vi "Routine.vi"(11 "Base Event in":refnum<class "Base Event.lvclass">) -> (3 "Base Event out":refnum<class "Base Event.lvclass">)   [LabVIEW 2021, in "jettl.lvlib" / "Base Event.lvlib" / "Base Event.lvclass"]
uses:
  Base Event.lvclass
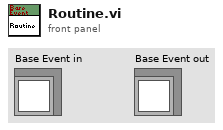
[diagram p1: front panel]
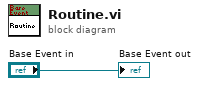
[diagram p0: block diagram]
diagram:
  "Base Event out" <- "Base Event in"
